vi "Show Windows(異常發生).vi"(8 "error in (no error)":errorcluster, 10 "Reset":bool caption="確認按鈕", 11 "String":string) -> (0 "error out":errorcluster)   [LabVIEW 2015]
panel:
  out "String 2":string
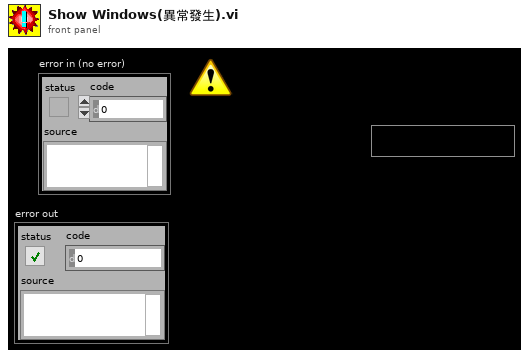
[diagram p1: front panel]
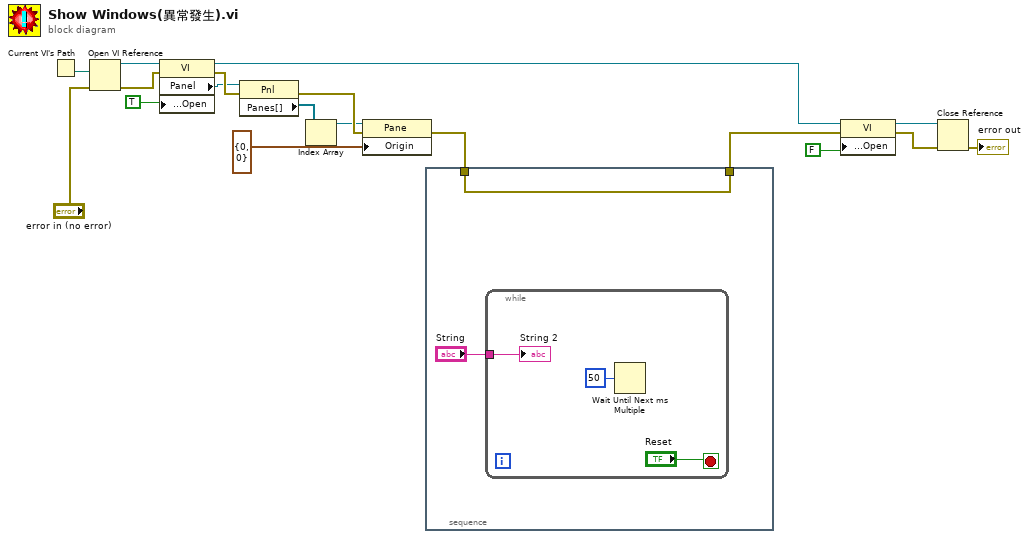
[diagram p0: block diagram]
diagram:
  n1 = Current VI's Path() -> (path=w16:path)
  n2 = Open VI Reference(vi path=w16, error in (no error)="error in (no error)") -> (vi reference=w10:refnum<vi>, error out=w11:errorcluster)  [unwired: 4 in]
  n3 = property class="VI"(reference=w10, error in=w11, "Front Panel.Open"=TRUE ("Front Panel Window:Open")) -> (reference out=w7:refnum<vi>, error out=w17:errorcluster, "Panel"=w15:refnum<vi>)
  n4 = property class="Pnl"(reference=w15, error in=w17) -> (error out=w18:errorcluster, "Panes[]"=w12:refnum<vi>[])  [unwired: 1 out]
  n5 = Index Array(array=w12) -> (element=w13:refnum<vi>)  [unwired: 1 in]
  n6 = property class="Pane"(reference=w13, error in=w18, "Origin"=cluster{"Horizontal":i16, "Vertical":i16} {"Horizontal"=0, "Vertical"=0}) -> (error out=w8:errorcluster)  [unwired: 1 out]
  n7 = stacked-sequence {
    tunnel: [w20] -> w4
    tunnel: w8 -> [w20]
    frame #0 {
      n8 = while {
        tunnel: "String" -> [w21]
        stop <- "Reset" stop-if-true
        n9 = Wait Until Next ms Multiple(millisecond multiple=u32 50) -> ()  [unwired: 1 out]
        "String 2" <- w21
      }
    }
  }
  n10 = property class="VI"(reference=w7, error in=w4, "Front Panel.Open"=FALSE ("Front Panel Window:Open")) -> (reference out=w6:refnum<vi>, error out=w3:errorcluster)
  n11 = Close Reference(reference=w6, error in (no error)=w3) -> (error out=→"error out":errorcluster)
